vi "open camera.vi"(8 "error in (no error)":errorcluster, 9 "Camera Settings":path, 10 "identifier":string, 11 "driver":T2) -> (0 "error out":errorcluster, 3 "Camera":T1)   [LabVIEW 2024, in "Vision.lvlib"]
uses:
  Vision.lvlib
  camera driver.ctl
  camera.ctl
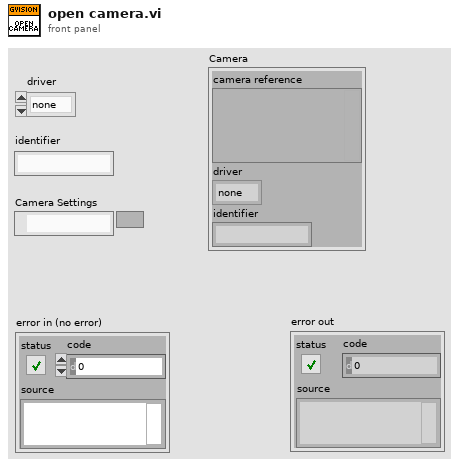
[diagram p1: front panel]
types:
  T1 = typedef "Vision.lvlib/camera.ctl" = cluster{"camera reference":variant, "driver":T2, "identifier":string}
  T2 = typedef "Vision.lvlib/camera driver.ctl" = enum16{"none", "ueye", "wmf", "imaqdx"}
  T3 = typedef "IMAQdx.ctl" = refnum<k21>
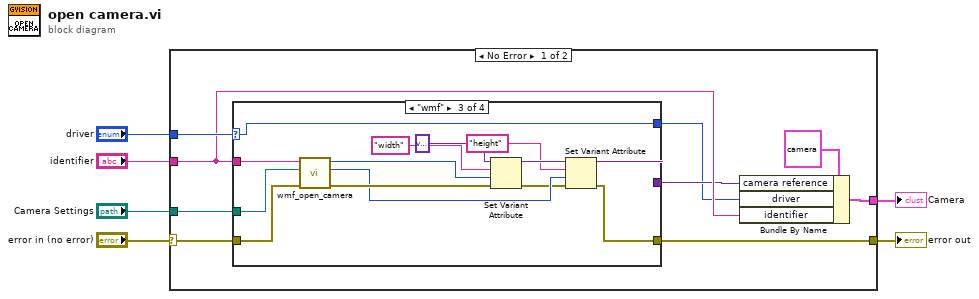
[diagram p0: block diagram]
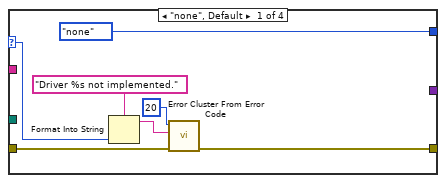
[diagram p2: hidden frame]
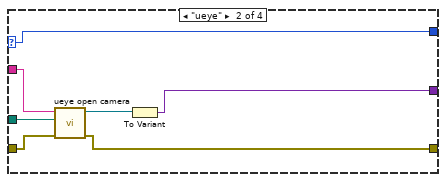
[diagram p3: hidden frame]
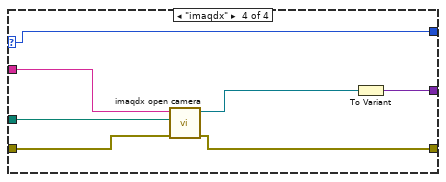
[diagram p4: hidden frame]
diagram:
  n1 = case shown="No Error" "error in (no error)" {
    selector: "error in (no error)" -> [w14 w51]
    tunnel: [w8 w51] -> w5
    tunnel: "driver" -> [w11 _]
    tunnel: "identifier" -> [w10 _]
    tunnel: "Camera Settings" -> [w15 _]
    tunnel: [w12 _] -> w1
    frame No Error {
      n2 = case shown="\"wmf\"" w11 {
        selector: w11 -> [w18 w29 w41 w50]
        tunnel: w10 -> [_ w27 w43 w49]
        tunnel: w15 -> [_ w28 w40 w48]
        tunnel: w14 -> [w21 w26 w42 w47]
        tunnel: [_ w23 w30 w44] -> w9
        tunnel: [w20 w24 w31 w46] -> w8
        tunnel: [camera_driver."none" ("driver") w29 w41 w50] -> w7
        frame "none", Default {
          n3 = Format Into String(format string="Driver %s not implemented.", w18) -> (resulting string=w17:string)  [unwired: 2 in, 1 out]
          n4 = call <vilib>:"Error Cluster From Error Code.vi"("error in (no error)"=w21, "error message (\"\")"=w17, "error code (0)"=20) -> ("error out"=w20:errorcluster)  [unwired: 6 in]
        }
        frame "ueye" {
          n5 = call "ueye open camera.vi"("error in (no error)"=w26, "Camera Settings"=w28, "identifier"=w27) -> ("error out"=w24:errorcluster, "Camera reference out"=w25:refnum<k24>)  [unwired: 7 in]
          n6 = To Variant(anything=w25) -> (Variant=w23:variant)
        }
        frame "wmf" {
          n7 = call "wmf_open_camera.vi"("error in (no error)"=w42, "Config path"=w40, "camera_name"=w43) -> ("error out"=w38:errorcluster, "height"=w34:i32, "width"=w36:i32)  [unwired: 6 in]
          n8 = Set Variant Attribute(Variant=variant, name="width", value=w36, error in=w38) -> (Variant out=w35:variant, error out=w32:errorcluster)  [unwired: 1 out]
          n9 = Set Variant Attribute(Variant=w35, name="height", value=w34, error in=w32) -> (Variant out=w30:variant, error out=w31:errorcluster)  [unwired: 1 out]
        }
        frame "imaqdx" {
          n10 = call "imaqdx open camera.vi"("error in (no error)"=w47, "Config File"=w48, "identifier"=w49) -> ("error out"=w46:errorcluster, "Session Out"=w45:T3)  [unwired: 7 in]
          n11 = To Variant(anything=w45) -> (Variant=w44:variant)
        }
      }
      n12 = Bundle By Name(cluster=T1 {"camera reference"=variant, "driver"=enum."none", "identifier"=""}, "camera reference"=w9, "driver"=w7, "identifier"=w10) -> (w12:T1)
    }
    frame Error {
    }
  }
  "error out" <- w5
  "Camera" <- w1
